vi "Write SP.vi"(8 "error in (no error)":errorcluster, 10 "SP":dbl, 11 "Generic Init CVT Message in":refnum<class "Generic Init CVT Message.lvclass">) -> (0 "error out":errorcluster, 3 "Generic Init CVT Message out":refnum<class "Generic Init CVT Message.lvclass">)   [LabVIEW 2014, in "DAQ Device.lvlib" / "Generic Init CVT Message.lvclass"]
uses:
  Generic Init CVT Message.lvclass
  Generic Init CVT Message.lvclass/Generic Init CVT Message.ctl
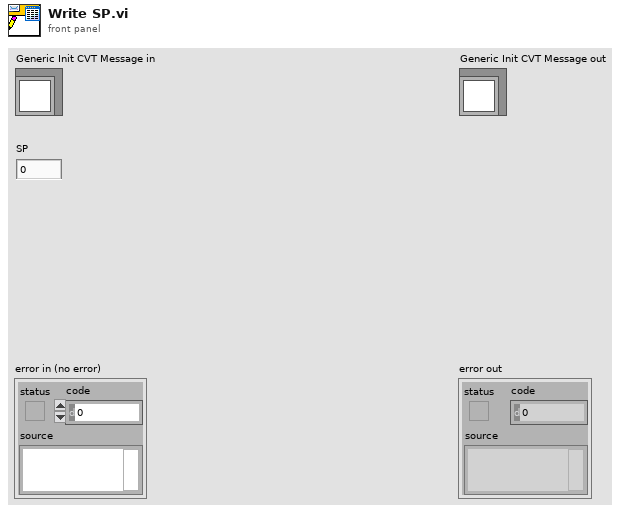
[diagram p1: front panel]
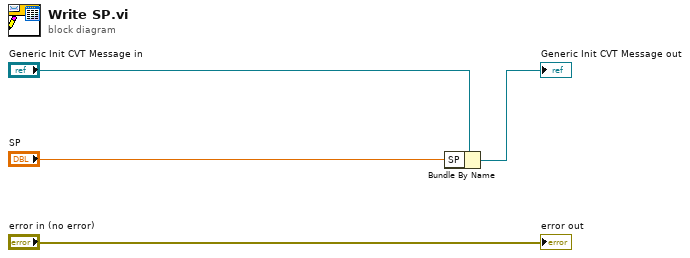
[diagram p0: block diagram]
diagram:
  n1 = Bundle By Name(cluster="Generic Init CVT Message in", "SP"="SP") -> (→"Generic Init CVT Message out":refnum<class "Generic Init CVT Message.lvclass">)
  "error out" <- "error in (no error)"
